vi "调用百度AI进行文字识别.vi"() -> ()   [LabVIEW 2019]
panel:
  out "x-y":u32
  out "子字符串之后":string
  out "new picture":picture caption="新图片"
  in  "路径":path
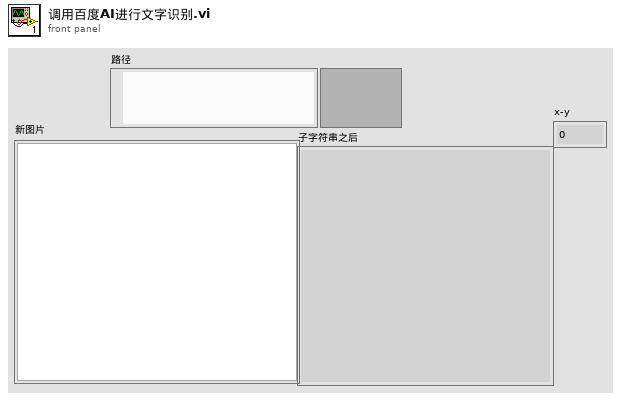
[diagram p1: front panel]
types:
  T1 = typedef "imagedata.ctl" = cluster{"image type":i32, "image depth":i32, "image":u8[], "mask":u8[], "colors":u32[], "Rectangle":cluster{"left":i16, "top":i16, "right":i16, "bottom":i16}}
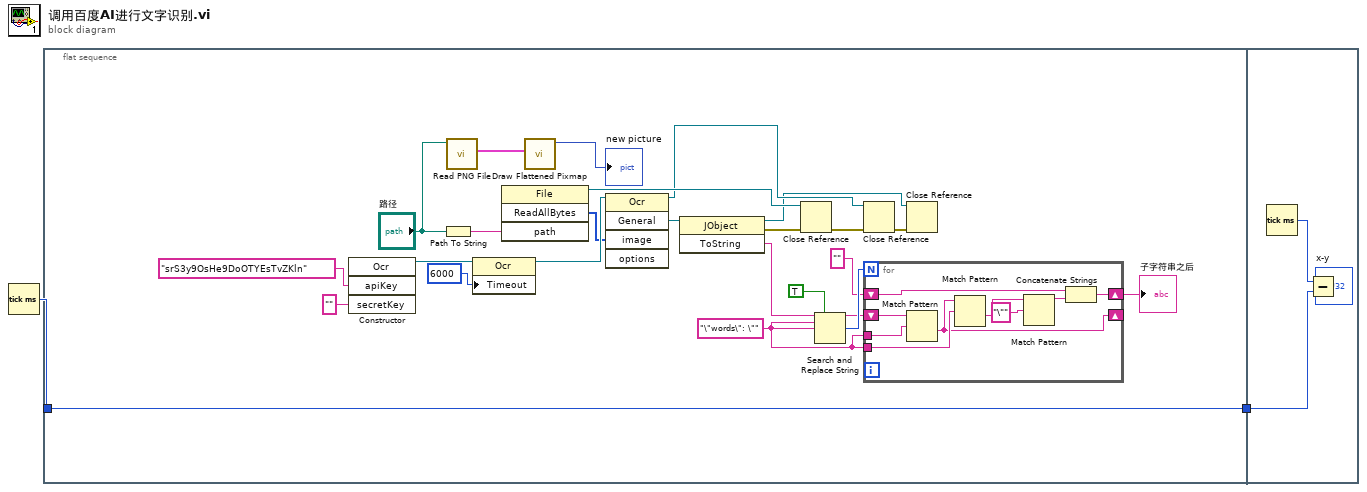
[diagram p0: block diagram]
diagram:
  n1 = Tick Count (ms)() -> (millisecond timer value=w2:u32)
  n2 = flat-sequence {
    tunnel: w2 -> [w3]
    tunnel: [w3] -> w1
    tunnel: w1 -> [w38]
    frame #0 {
      w12 = "\"words\": \"" ("正则表达式")
      n3 = constructor class="Ocr"("apiKey"="srS3y9OsHe9DoOTYEsTvZKln", "secretKey"="") -> (reference out=w25:refnum<k24>)  [unwired: 3 in, 4 out]
      n4 = Path To String(path="路径") -> (string=w21:string)
      n5 = call <vilib>:"Read PNG File.vi"("path to PNG file"="路径") -> ("image data"=w19:T1)  [unwired: 8 in, 2 out]
      n6 = property on="属性节点" class="Ocr"(reference=w25, "Timeout"=6000) -> (reference out=w23:refnum<k24>)  [unwired: 1 in, 1 out]
      n7 = invoke on="调用节点" class="File" method="ReadAllBytes"("path"=w21) -> (reference out=w7:refnum<k24>, "ReadAllBytes"=w20:u8[])  [unwired: 3 in, 2 out]
      n8 = call <vilib>:"Draw Flattened Pixmap.vi"("image data"=w19) -> ("new picture"=→"new picture":picture)  [unwired: 8 in]
      n9 = invoke on="调用节点" class="Ocr" method="General"(reference=w23, "image"=w20) -> (reference out=w6:refnum<k24>, "General"=w22:refnum<k24>)  [unwired: 3 in, 3 out]
      n10 = invoke on="调用节点" class="JObject" method="ToString"(reference=w22) -> (reference out=w5:refnum<k24>, error out=w4:errorcluster, "ToString"=w16:string)  [unwired: 2 in]
      n11 = Close Reference(reference=w7, error in (no error)=w4) -> (error out=w8:errorcluster)
      n12 = Search and Replace String(replace all?=TRUE ("替换全部？(F)"), input string=w16, search string=w12, replace string=w12) -> (result string=w13:string, number of replacements=w14:i32)  [unwired: 4 in, 2 out]
      n13 = Close Reference(reference=w6, error in (no error)=w8) -> (error out=w9:errorcluster)
      n14 = for {
        N: w14 -> [_]
        shift-right: [w31] -> _
        shift-left: w13 -> [w36]
        tunnel: w12 -> [w35]
        tunnel: w12 -> [w32]
        shift-right: [w28] -> w10
        shift-left: "" ("result string") -> [w29]
        n15 = Match Pattern(string=w36, regular expression=w35) -> (after substring=w31:string)  [unwired: 1 in, 3 out]
        n16 = Match Pattern(string=w31, regular expression=w32) -> (after substring=w34:string)  [unwired: 1 in, 3 out]
        n17 = Match Pattern(string=w34, regular expression="\"" ("正则表达式")) -> (before substring=w30:string)  [unwired: 1 in, 3 out]
        n18 = Concatenate Strings(w29, w30) -> (w28:string)
      }
      "子字符串之后" <- w10
      n19 = Close Reference(reference=w5, error in (no error)=w9) -> ()  [unwired: 1 out]
    }
    frame #1 {
      n20 = Tick Count (ms)() -> (millisecond timer value=w39:u32)
      n21 = Subtract(x=w39, y=w38) -> (x-y=→"x-y":u32)
    }
  }
